vi "setRunToDocument.vi"(8 "error in (no error)":errorcluster, 11 "xwpfRun.Figure in":refnum<class "xwpfRun.Figure.lvclass">) -> (0 "error out":errorcluster, 3 "xwpfRun.Figure out":refnum<class "xwpfRun.Figure.lvclass">)   [LabVIEW 2017, in "Word_Specific.lvlib" / "xwpfRun.Figure.lvclass"]
uses:
  xwpfRun.Figure.lvclass
  C:/Users/Neo/Desktop/Dev_Tools_BR/LabVIEW_NPOI/src/LabVIEW NPOI/xwpfRun/xwpfRun.lvclass
  xwpfRun/xwpfRun.lvclass/xwpfRun.ctl
  xwpfRun.Figure.lvclass/xwpfRun.Figure.ctl
  C:/Users/Neo/Desktop/Dev_Tools_BR/LabVIEW_NPOI/src/lib/NPOI 2.1.1/NPOI.OOXML.dll
  lib/NPOI 2.1.1/NPOI.OOXML.dll
  xwpfRun/Get Run Ref.vi
  xwpfRun/xwpfRun.lvclass
  Support/File Stream/File Stream.lvlib
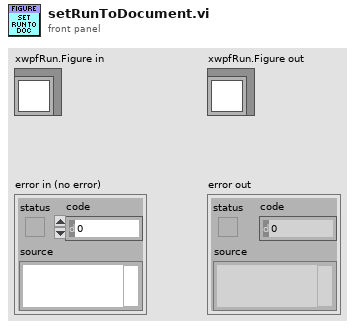
[diagram p1: front panel]
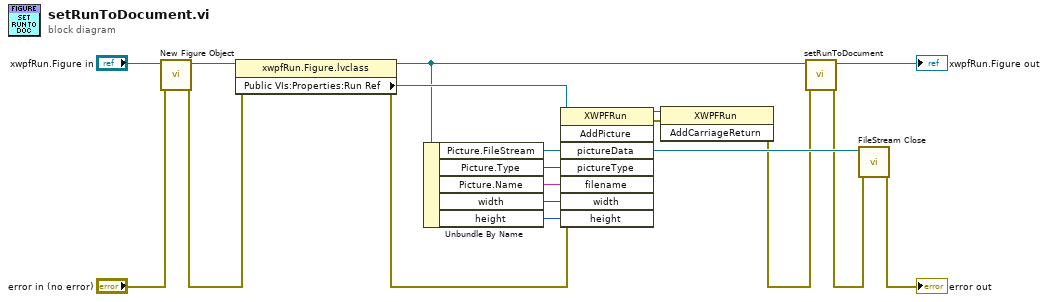
[diagram p0: block diagram]
diagram:
  n1 = call "New Figure Object.vi"("error in (no error)"="error in (no error)", "xwpfRun.Figure in"="xwpfRun.Figure in") -> ("error out"=w13:errorcluster, "xwpfRun.Figure out"=w12:refnum<class "xwpfRun.Figure.lvclass">)  [unwired: 8 in]
  n2 = property class="xwpfRun.Figure.lvclass"(reference=w12, error in=w13) -> (reference out=w7:refnum<class "xwpfRun.Figure.lvclass">, error out=w16:errorcluster, "Public VIs:Properties:Run Ref"=w18:refnum<k24>)
  n3 = Unbundle By Name(w7) -> ("Picture.FileStream"=w6:refnum<k24>, "Picture.Type"=w11:i32, "Picture.Name"=w10:string, "width"=w9:i32, "height"=w8:i32)
  n4 = invoke class="XWPFRun" method="AddPicture"(reference=w18, error in=w16, "pictureData"=w6, "pictureType"=w11, "filename"=w10, "width"=w9, "height"=w8) -> (reference out=w2:refnum<k24>, error out=w3:errorcluster)  [unwired: 1 in, 6 out]
  n5 = invoke class="XWPFRun" method="AddCarriageReturn"(reference=w2, error in=w3) -> (error out=w1:errorcluster)  [unwired: 1 in, 2 out]
  n6 = call-parent "setRunToDocument.vi"("error in (no error)"=w1, "xwpfRun in"=w7) -> ("error out"=w5:errorcluster, "xwpfRun out"=→"xwpfRun.Figure out":refnum<class "xwpfRun.Figure.lvclass">)  [unwired: 8 in]
  n7 = call "FileStream Close.vi"("error in (no error)"=w5, "reference"=w6) -> ("error out"=→"error out":errorcluster)  [unwired: 9 in]
